vi "Maze.vi"() -> ()   [LabVIEW 2015]
panel:
  out "Message":string
  in  "Reset":bool
  out "Coordinates":dbl
  in  "Down":bool
  in  "Up":bool
  in  "Right":bool
  in  "Left":bool
  out "Finish":bool
  out "Start":bool
  out "44":bool
  out "34":bool
  out "24":bool
  out "14":bool
  out "43":bool
  out "33":bool
  out "23":bool
  out "13":bool
  out "42":bool
  out "32":bool
  out "22":bool
  out "12":bool
  out "41":bool
  out "31":bool
  out "21":bool
  out "11":bool
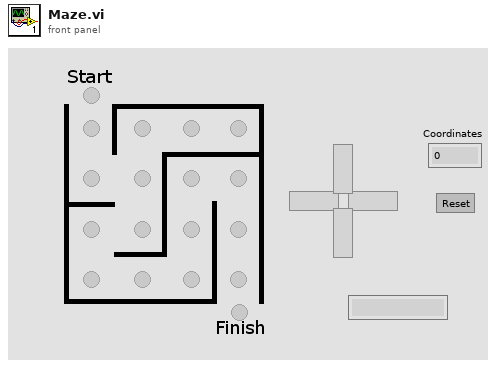
[diagram p1: front panel]
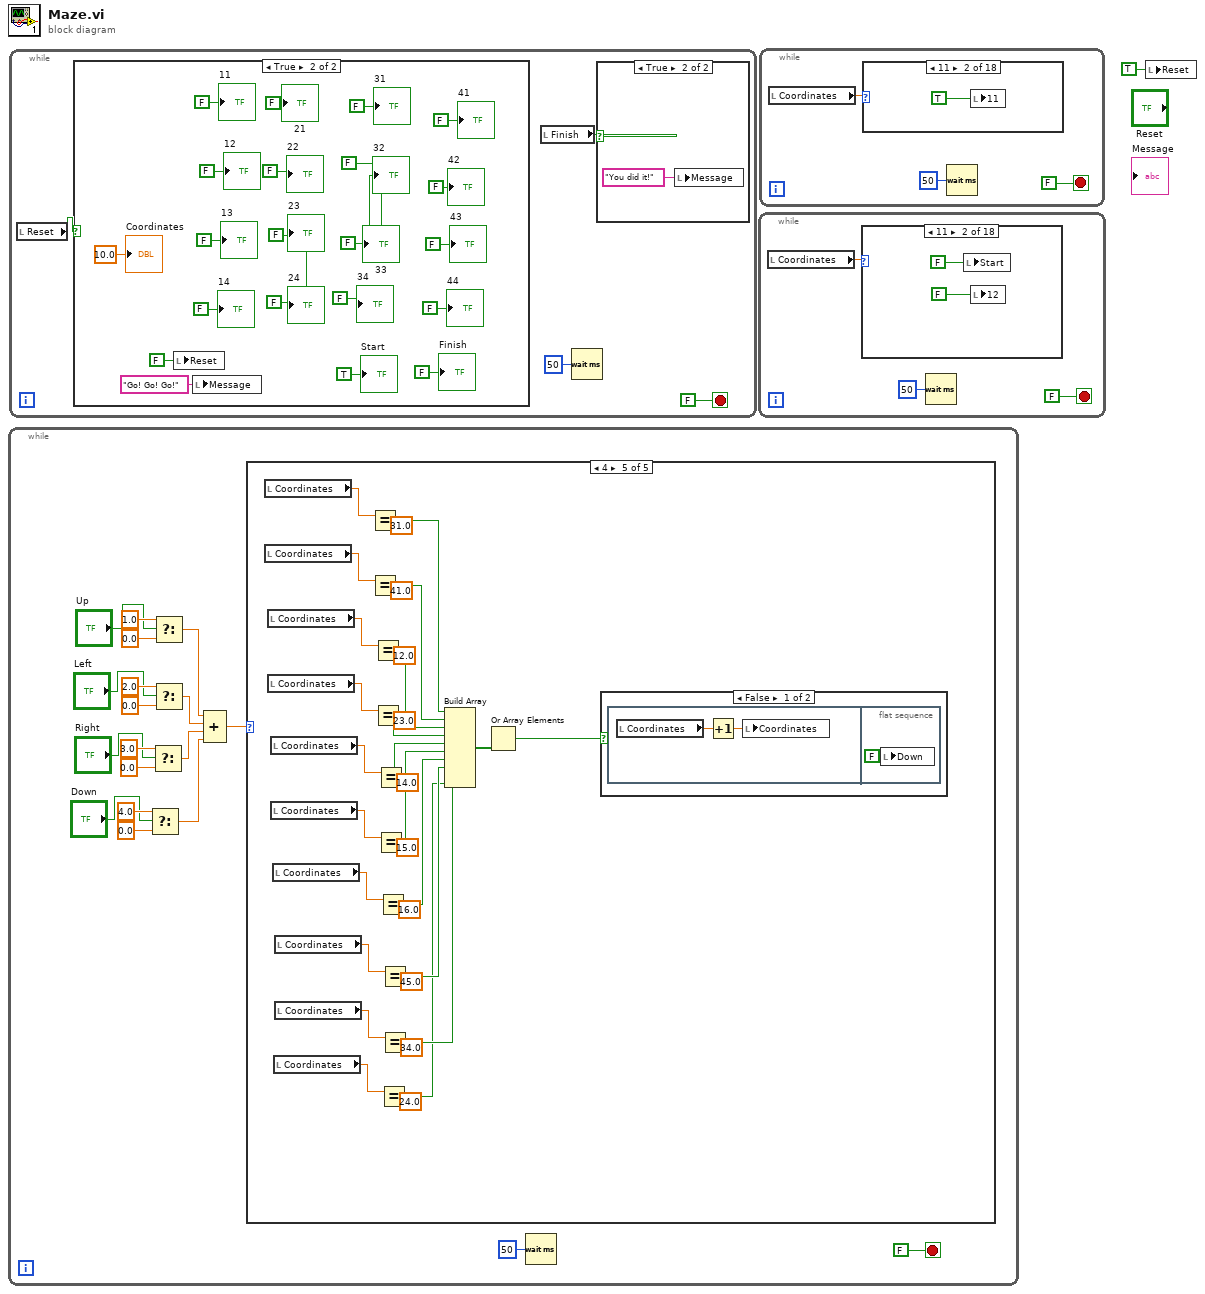
[diagram p0: block diagram]
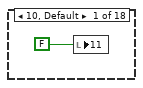
[diagram p2: hidden frame]
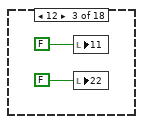
[diagram p3: hidden frame]
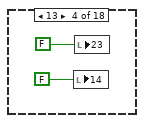
[diagram p4: hidden frame]
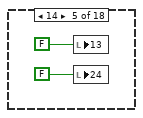
[diagram p5: hidden frame]
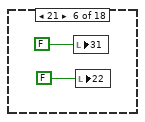
[diagram p6: hidden frame]
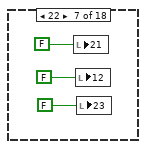
[diagram p7: hidden frame]
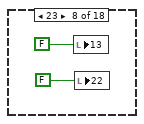
[diagram p8: hidden frame]
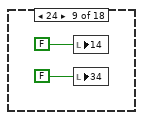
[diagram p9: hidden frame]
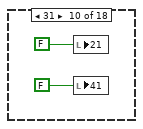
[diagram p10: hidden frame]
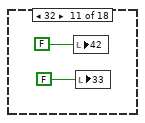
[diagram p11: hidden frame]
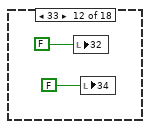
[diagram p12: hidden frame]
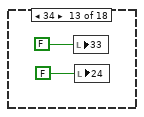
[diagram p13: hidden frame]
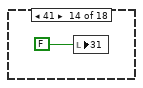
[diagram p14: hidden frame]
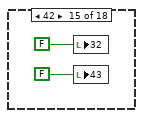
[diagram p15: hidden frame]
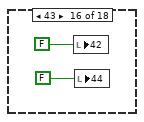
[diagram p16: hidden frame]
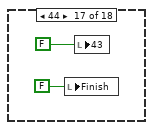
[diagram p17: hidden frame]
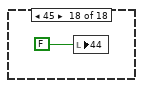
[diagram p18: hidden frame]
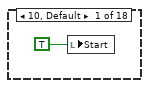
[diagram p19: hidden frame]
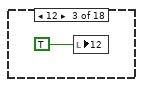
[diagram p20: hidden frame]
diagram:
  n1 = while {
    stop <- FALSE stop-if-true
    n2 = Select(t=4.0, s="Down", f=0.0) -> (s? t:f=w8:dbl)
    n3 = Select(t=3.0, s="Right", f=0.0) -> (s? t:f=w5:dbl)
    n4 = Select(t=1.0, s="Up", f=0.0) -> (s? t:f=w7:dbl)
    n5 = Select(t=2.0, s="Left", f=0.0) -> (s? t:f=w6:dbl)
    n6 = Compound Arithmetic op=ADD(w7, w6, w5, w8) -> (w4:dbl)
    n7 = case shown="4" w4 {
      frame 0, Default {
      }
      frame 1 {
        n8 = local read "Coordinates"() -> (w46:dbl)
        n9 = local read "Coordinates"() -> (w43:dbl)
        n10 = local read "Coordinates"() -> (w42:dbl)
        n11 = local read "Coordinates"() -> (w39:dbl)
        n12 = local read "Coordinates"() -> (w35:dbl)
        n13 = local read "Coordinates"() -> (w38:dbl)
        n14 = local read "Coordinates"() -> (w34:dbl)
        n15 = local read "Coordinates"() -> (w31:dbl)
        n16 = Equal?(x=w46, y=10.0) -> (x = y?=w30:bool)
        n17 = Equal?(x=w43, y=21.0) -> (x = y?=w29:bool)
        n18 = Equal?(x=w42, y=31.0) -> (x = y?=w28:bool)
        n19 = Equal?(x=w39, y=41.0) -> (x = y?=w27:bool)
        n20 = Equal?(x=w35, y=32.0) -> (x = y?=w26:bool)
        n21 = Equal?(x=w38, y=42.0) -> (x = y?=w25:bool)
        n22 = Equal?(x=w34, y=13.0) -> (x = y?=w24:bool)
        n23 = Equal?(x=w31, y=24.0) -> (x = y?=w23:bool)
        n24 = Build Array(w30, w29, w28, w27, w26, w25, w24, w23) -> (w22:bool[])
        n25 = Or Array Elements(Boolean array=w22) -> (logical OR=w21:bool)
        n26 = case shown="False" w21 {
          frame False {
            n27 = flat-sequence {
              frame #0 {
                n28 = local read "Coordinates"() -> (w48:dbl)
                n29 = Decrement(x=w48) -> (x-1=w47:dbl)
                n30 = local write "Coordinates"(w47) -> ()
              }
              frame #1 {
                n31 = local write "Up"(FALSE ("Up")) -> ()
              }
            }
          }
          frame True {
            n32 = local write "Up"(FALSE ("Up")) -> ()
          }
        }
      }
      frame 2 {
        n33 = local read "Coordinates"() -> (w85:dbl)
        n34 = local read "Coordinates"() -> (w82:dbl)
        n35 = local read "Coordinates"() -> (w81:dbl)
        n36 = local read "Coordinates"() -> (w78:dbl)
        n37 = local read "Coordinates"() -> (w52:dbl)
        n38 = local read "Coordinates"() -> (w74:dbl)
        n39 = local read "Coordinates"() -> (w77:dbl)
        n40 = local read "Coordinates"() -> (w73:dbl)
        n41 = local read "Coordinates"() -> (w70:dbl)
        n42 = local read "Coordinates"() -> (w56:dbl)
        n43 = local read "Coordinates"() -> (w59:dbl)
        n44 = Equal?(x=w85, y=10.0) -> (x = y?=w69:bool)
        n45 = Equal?(x=w82, y=11.0) -> (x = y?=w68:bool)
        n46 = Equal?(x=w81, y=12.0) -> (x = y?=w67:bool)
        n47 = Equal?(x=w78, y=13.0) -> (x = y?=w66:bool)
        n48 = Equal?(x=w52, y=45.0) -> (x = y?=w51:bool)
        n49 = Equal?(x=w74, y=14.0) -> (x = y?=w65:bool)
        n50 = Equal?(x=w77, y=21.0) -> (x = y?=w64:bool)
        n51 = Equal?(x=w73, y=32.0) -> (x = y?=w63:bool)
        n52 = Equal?(x=w70, y=33.0) -> (x = y?=w62:bool)
        n53 = Equal?(x=w56, y=43.0) -> (x = y?=w55:bool)
        n54 = Equal?(x=w59, y=44.0) -> (x = y?=w54:bool)
        n55 = Build Array(w69, w68, w67, w66, w65, w64, w63, w62, w55, w54, w51) -> (w61:bool[])
        n56 = Or Array Elements(Boolean array=w61) -> (logical OR=w60:bool)
        n57 = case shown="False" w60 {
          frame False {
            n58 = flat-sequence {
              frame #0 {
                n59 = local read "Coordinates"() -> (w87:dbl)
                n60 = Subtract(x=w87, y=10.0) -> (x-y=w88:dbl)
                n61 = local write "Coordinates"(w88) -> ()
              }
              frame #1 {
                n62 = local write "Left"(FALSE ("Up")) -> ()
              }
            }
          }
          frame True {
            n63 = local write "Left"(FALSE ("Up")) -> ()
          }
        }
      }
      frame 3 {
        n64 = local read "Coordinates"() -> (w125:dbl)
        n65 = local read "Coordinates"() -> (w122:dbl)
        n66 = local read "Coordinates"() -> (w121:dbl)
        n67 = local read "Coordinates"() -> (w118:dbl)
        n68 = local read "Coordinates"() -> (w92:dbl)
        n69 = local read "Coordinates"() -> (w114:dbl)
        n70 = local read "Coordinates"() -> (w117:dbl)
        n71 = local read "Coordinates"() -> (w113:dbl)
        n72 = local read "Coordinates"() -> (w110:dbl)
        n73 = local read "Coordinates"() -> (w96:dbl)
        n74 = local read "Coordinates"() -> (w99:dbl)
        n75 = Equal?(x=w125, y=10.0) -> (x = y?=w109:bool)
        n76 = Equal?(x=w122, y=11.0) -> (x = y?=w108:bool)
        n77 = Equal?(x=w121, y=41.0) -> (x = y?=w107:bool)
        n78 = Equal?(x=w118, y=22.0) -> (x = y?=w106:bool)
        n79 = Equal?(x=w92, y=45.0) -> (x = y?=w91:bool)
        n80 = Equal?(x=w114, y=42.0) -> (x = y?=w105:bool)
        n81 = Equal?(x=w117, y=23.0) -> (x = y?=w104:bool)
        n82 = Equal?(x=w113, y=33.0) -> (x = y?=w103:bool)
        n83 = Equal?(x=w110, y=43.0) -> (x = y?=w102:bool)
        n84 = Equal?(x=w96, y=34.0) -> (x = y?=w95:bool)
        n85 = Equal?(x=w99, y=44.0) -> (x = y?=w94:bool)
        n86 = Build Array(w109, w108, w107, w106, w105, w104, w103, w102, w95, w94, w91) -> (w101:bool[])
        n87 = Or Array Elements(Boolean array=w101) -> (logical OR=w100:bool)
        n88 = case shown="False" w100 {
          frame False {
            n89 = flat-sequence {
              frame #0 {
                n90 = local read "Coordinates"() -> (w127:dbl)
                n91 = Add(x=w127, y=10.0) -> (x+y=w128:dbl)
                n92 = local write "Coordinates"(w128) -> ()
              }
              frame #1 {
                n93 = local write "Right"(FALSE ("Up")) -> ()
              }
            }
          }
          frame True {
            n94 = local write "Right"(FALSE ("Up")) -> ()
          }
        }
      }
      frame 4 {
        n95 = local read "Coordinates"() -> (w162:dbl)
        n96 = local read "Coordinates"() -> (w159:dbl)
        n97 = local read "Coordinates"() -> (w158:dbl)
        n98 = local read "Coordinates"() -> (w155:dbl)
        n99 = local read "Coordinates"() -> (w151:dbl)
        n100 = local read "Coordinates"() -> (w154:dbl)
        n101 = local read "Coordinates"() -> (w150:dbl)
        n102 = local read "Coordinates"() -> (w132:dbl)
        n103 = local read "Coordinates"() -> (w138:dbl)
        n104 = local read "Coordinates"() -> (w136:dbl)
        n105 = Equal?(x=w162, y=31.0) -> (x = y?=w148:bool)
        n106 = Equal?(x=w159, y=41.0) -> (x = y?=w147:bool)
        n107 = Equal?(x=w158, y=12.0) -> (x = y?=w146:bool)
        n108 = Equal?(x=w155, y=23.0) -> (x = y?=w145:bool)
        n109 = Equal?(x=w151, y=14.0) -> (x = y?=w144:bool)
        n110 = Equal?(x=w154, y=15.0) -> (x = y?=w143:bool)
        n111 = Equal?(x=w150, y=16.0) -> (x = y?=w142:bool)
        n112 = Equal?(x=w132, y=24.0) -> (x = y?=w131:bool)
        n113 = Equal?(x=w138, y=45.0) -> (x = y?=w137:bool)
        n114 = Equal?(x=w136, y=34.0) -> (x = y?=w134:bool)
        n115 = Build Array(w148, w147, w146, w145, w144, w143, w142, w137, w134, w131) -> (w141:bool[])
        n116 = Or Array Elements(Boolean array=w141) -> (logical OR=w140:bool)
        n117 = case shown="False" w140 {
          frame False {
            n118 = flat-sequence {
              frame #0 {
                n119 = local read "Coordinates"() -> (w164:dbl)
                n120 = Increment(x=w164) -> (x+1=w163:dbl)
                n121 = local write "Coordinates"(w163) -> ()
              }
              frame #1 {
                n122 = local write "Down"(FALSE ("Up")) -> ()
              }
            }
          }
          frame True {
            n123 = local write "Down"(FALSE ("Up")) -> ()
          }
        }
      }
    }
    n124 = Wait (ms)(milliseconds to wait=u32 50) -> ()  [unwired: 1 out]
  }
  n125 = while {
    stop <- FALSE stop-if-true
    n126 = local read "Reset"() -> (w170:bool)
    n127 = case shown="True" w170 {
      frame False {
      }
      frame True {
        n128 = local write "Reset"(FALSE ("Reset")) -> ()
        n129 = local write "Message"("Go! Go! Go!") -> ()
        "11" <- FALSE ("Boolean")
        "21" <- FALSE ("Boolean 2")
        "31" <- FALSE ("Boolean 3")
        "41" <- FALSE ("Boolean 4")
        "12" <- FALSE ("Boolean 5")
        "22" <- FALSE ("Boolean 6")
        "32" <- FALSE ("Boolean 7")
        "42" <- FALSE ("Boolean 8")
        "13" <- FALSE ("Boolean 9")
        "23" <- FALSE ("Boolean 10")
        "33" <- FALSE ("Boolean 11")
        "43" <- FALSE ("Boolean 12")
        "14" <- FALSE ("Boolean 13")
        "24" <- FALSE ("Boolean 14")
        "34" <- FALSE ("Boolean 15")
        "44" <- FALSE ("Boolean 16")
        "Start" <- TRUE ("Start")
        "Finish" <- FALSE ("Finish")
        "Coordinates" <- 10.0 ("Coordinates")
      }
    }
    n130 = local read "Finish"() -> (w167:bool)
    n131 = Wait (ms)(milliseconds to wait=u32 50) -> ()  [unwired: 1 out]
    n132 = case shown="True" w167 {
      frame False {
      }
      frame True {
        n133 = local write "Message"("You did it!") -> ()
      }
    }
  }
  n134 = while {
    stop <- FALSE stop-if-true
    n135 = local read "Coordinates"() -> (w195:dbl)
    n136 = case shown="11" w195 {
      frame 10, Default {
        n137 = local write "11"(FALSE ("Boolean")) -> ()
      }
      frame 11 {
        n138 = local write "Start"(FALSE ("Boolean")) -> ()
        n139 = local write "12"(FALSE ("Boolean")) -> ()
      }
      frame 12 {
        n140 = local write "11"(FALSE ("Boolean")) -> ()
        n141 = local write "22"(FALSE ("Boolean")) -> ()
      }
      frame 13 {
        n142 = local write "14"(FALSE ("Boolean")) -> ()
        n143 = local write "23"(FALSE ("Boolean")) -> ()
      }
      frame 14 {
        n144 = local write "13"(FALSE ("Boolean")) -> ()
        n145 = local write "24"(FALSE ("Boolean")) -> ()
      }
      frame 21 {
        n146 = local write "31"(FALSE ("Boolean")) -> ()
        n147 = local write "22"(FALSE ("Boolean")) -> ()
      }
      frame 22 {
        n148 = local write "21"(FALSE ("Boolean")) -> ()
        n149 = local write "12"(FALSE ("Boolean")) -> ()
        n150 = local write "23"(FALSE ("Boolean")) -> ()
      }
      frame 23 {
        n151 = local write "13"(FALSE ("Boolean")) -> ()
        n152 = local write "22"(FALSE ("Boolean")) -> ()
      }
      frame 24 {
        n153 = local write "14"(FALSE ("Boolean")) -> ()
        n154 = local write "34"(FALSE ("Boolean")) -> ()
      }
      frame 31 {
        n155 = local write "21"(FALSE ("Boolean")) -> ()
        n156 = local write "41"(FALSE ("Boolean")) -> ()
      }
      frame 32 {
        n157 = local write "42"(FALSE ("Boolean")) -> ()
        n158 = local write "33"(FALSE ("Boolean")) -> ()
      }
      frame 33 {
        n159 = local write "32"(FALSE ("Boolean")) -> ()
        n160 = local write "34"(FALSE ("Boolean")) -> ()
      }
      frame 34 {
        n161 = local write "33"(FALSE ("Boolean")) -> ()
        n162 = local write "24"(FALSE ("Boolean")) -> ()
      }
      frame 41 {
        n163 = local write "31"(FALSE ("Boolean")) -> ()
      }
      frame 42 {
        n164 = local write "32"(FALSE ("Boolean")) -> ()
        n165 = local write "43"(FALSE ("Boolean")) -> ()
      }
      frame 43 {
        n166 = local write "42"(FALSE ("Boolean")) -> ()
        n167 = local write "44"(FALSE ("Boolean")) -> ()
      }
      frame 44 {
        n168 = local write "Finish"(FALSE ("Boolean")) -> ()
        n169 = local write "43"(FALSE ("Boolean")) -> ()
      }
      frame 45 {
        n170 = local write "44"(FALSE ("Boolean")) -> ()
      }
    }
    n171 = Wait (ms)(milliseconds to wait=u32 50) -> ()  [unwired: 1 out]
  }
  n172 = while {
    stop <- FALSE stop-if-true
    n173 = local read "Coordinates"() -> (w232:dbl)
    n174 = case shown="11" w232 {
      frame 10, Default {
        n175 = local write "Start"(TRUE ("Boolean")) -> ()
      }
      frame 11 {
        n176 = local write "11"(TRUE ("Boolean")) -> ()
      }
      frame 12 {
        n177 = local write "12"(TRUE ("Boolean")) -> ()
      }
      frame 13 {
        n178 = local write "13"(TRUE ("Boolean")) -> ()
      }
      frame 14 {
        n179 = local write "14"(TRUE ("Boolean")) -> ()
      }
      frame 21 {
        n180 = local write "21"(TRUE ("Boolean")) -> ()
      }
      frame 22 {
        n181 = local write "22"(TRUE ("Boolean")) -> ()
      }
      frame 23 {
        n182 = local write "23"(TRUE ("Boolean")) -> ()
      }
      frame 24 {
        n183 = local write "24"(TRUE ("Boolean")) -> ()
      }
      frame 31 {
        n184 = local write "31"(TRUE ("Boolean")) -> ()
      }
      frame 32 {
        n185 = local write "32"(TRUE ("Boolean")) -> ()
      }
      frame 33 {
        n186 = local write "33"(TRUE ("Boolean")) -> ()
      }
      frame 34 {
        n187 = local write "34"(TRUE ("Boolean")) -> ()
      }
      frame 41 {
        n188 = local write "41"(TRUE ("Boolean")) -> ()
      }
      frame 42 {
        n189 = local write "42"(TRUE ("Boolean")) -> ()
      }
      frame 43 {
        n190 = local write "43"(TRUE ("Boolean")) -> ()
      }
      frame 44 {
        n191 = local write "44"(TRUE ("Boolean")) -> ()
      }
      frame 45 {
        n192 = local write "Finish"(TRUE ("Boolean")) -> ()
      }
    }
    n193 = Wait (ms)(milliseconds to wait=u32 50) -> ()  [unwired: 1 out]
  }
  n194 = local write "Reset"(TRUE ("Reset")) -> ()
